vi "BMP180 Init.vi"(7 "I2C Channel":u8=1, 8 "error in (no error)":errorcluster, 9 "BMP180 Config Options":T1={"Mode"=enum."Ultra Low Power", "Cal Coefs"={"AC1"={"Addr:"=170, "Val:"=0}, "AC2"={"Addr:"=172, "Val:"=0}, "AC3"={"Addr:"=174, "Val:"=0}, "AC4"={"Addr:"=176, "Val:"=0}, "AC5"={"Addr:"=178, "Val:"=0}, "AC6"={"Addr:"=180, "Val:"=0}, "B1"={"Addr:"=182, "Val:"=0}, "B2"={"Addr:"=184, "Val:"=0}, "MB"={"Addr:"=186, "Val:"=0}, "MC"={"Addr:"=188, "Val:"=0}, "MD"={"Addr:"=190, "Val:"=0}}} {"Cal Coefs"."MD"."Val:" format="%04x"; "Cal Coefs"."MD"."Addr:" format="%02x"; "Cal Coefs"."MC"."Val:" format="%04x"; "Cal Coefs"."MC"."Addr:" format="%02x"; "Cal Coefs"."MB"."Val:" format="%04x"; "Cal Coefs"."MB"."Addr:" format="%02x"; "Cal Coefs"."B2"."Val:" format="%04x"; "Cal Coefs"."B2"."Addr:" format="%02x"; "Cal Coefs"."B1"."Val:" format="%04x"; "Cal Coefs"."B1"."Addr:" format="%02x"; "Cal Coefs"."AC6"."Val:" format="%04x"; "Cal Coefs"."AC6"."Addr:" format="%02x"; "Cal Coefs"."AC5"."Val:" format="%04x"; "Cal Coefs"."AC5"."Addr:" format="%02x"; "Cal Coefs"."AC4"."Val:" format="%04x"; "Cal Coefs"."AC4"."Addr:" format="%02x"; "Cal Coefs"."AC3"."Val:" format="%04x"; "Cal Coefs"."AC3"."Addr:" format="%02x"; "Cal Coefs"."AC2"."Val:" format="%04x"; "Cal Coefs"."AC2"."Addr:" format="%02x"; "Cal Coefs"."AC1"."Val:" format="%04x"; "Cal Coefs"."AC1"."Addr:" format="%02x"}, 10 "I2C Slave Address":u8=119 format="%.0x", 11 "LINX Resource in":T2) -> (0 "error out":errorcluster, 1 "BMP180 Config Options":T1 {"Cal Coefs"."MD"."Val:" format="%04x"; "Cal Coefs"."MD"."Addr:" format="%02x"; "Cal Coefs"."MC"."Val:" format="%04x"; "Cal Coefs"."MC"."Addr:" format="%02x"; "Cal Coefs"."MB"."Val:" format="%04x"; "Cal Coefs"."MB"."Addr:" format="%02x"; "Cal Coefs"."B2"."Val:" format="%04x"; "Cal Coefs"."B2"."Addr:" format="%02x"; "Cal Coefs"."B1"."Val:" format="%04x"; "Cal Coefs"."B1"."Addr:" format="%02x"; "Cal Coefs"."AC6"."Val:" format="%04x"; "Cal Coefs"."AC6"."Addr:" format="%02x"; "Cal Coefs"."AC5"."Val:" format="%04x"; "Cal Coefs"."AC5"."Addr:" format="%02x"; "Cal Coefs"."AC4"."Val:" format="%04x"; "Cal Coefs"."AC4"."Addr:" format="%02x"; "Cal Coefs"."AC3"."Val:" format="%04x"; "Cal Coefs"."AC3"."Addr:" format="%02x"; "Cal Coefs"."AC2"."Val:" format="%04x"; "Cal Coefs"."AC2"."Addr:" format="%02x"; "Cal Coefs"."AC1"."Val:" format="%04x"; "Cal Coefs"."AC1"."Addr:" format="%02x"}, 3 "LINX Resource out":T2)   [LabVIEW 2014]
uses:
  <vilib>/MakerHub/LINX/Private/Type Defs/LINX Ref.ctl
  <vilib>/MakerHub/LINX/Private/Type Defs/Platform.ctl
  <vilib>/MakerHub/LINX/Private/Type Defs/Interface.ctl
  <vilib>/MakerHub/LINX/Private/Device/Type Defs/LINX Device Config.ctl
  <vilib>/MakerHub/LINX/Private/Device/Type Defs/TCP Config.ctl
  <vilib>/MakerHub/LINX/Private/Device/Type Defs/Channels.ctl
  BMP180 Config Options.ctl
  <vilib>/MakerHub/LINX/Private/Local IO/LinxI2cWrite.vi
  <vilib>/MakerHub/LINX/Public/Utilities/Check Channel.vi
  <vilib>/myRIO/Instrument Drivers/Onboard IO/I2C/vis/Write.vi
  <vilib>/MakerHub/LINX/Private/Utilties/Generate Error.vi
  <vilib>/MakerHub/LINX/Private/Utilties/Channel FGVs/I2C Channels.vi
  <vilib>/Utility/error.llb/Error Cluster From Error Code.vi
  <vilib>/myRIO/Common/Instrument Driver Framework/myRIO v1.0/I2C/vis/myRIO v1.0 Write I2C.vi
  <vilib>/MakerHub/LINX/LMH-LINX.lvlib
  <vilib>/MakerHub/LINX/Private/Device/Device.lvlib
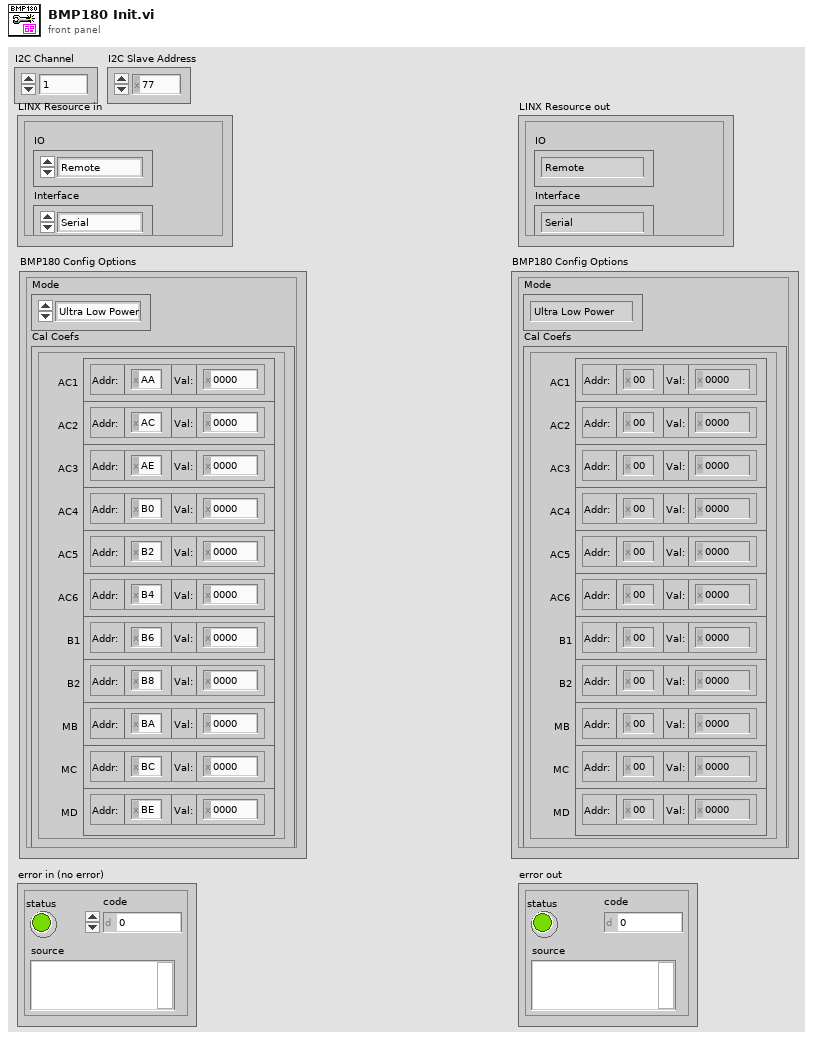
[diagram p1: front panel]
types:
  T1 = typedef "BMP180 Config Options.ctl" = cluster{"Mode":enum8{"Ultra Low Power", "Standard", "High Resolution", "Ultra High Resolution"}, "Cal Coefs":cluster{"AC1":cluster{"Addr:":u8, "Val:":u16}, "AC2":cluster{"Addr:":u8, "Val:":u16}, "AC3":cluster{"Addr:":u8, "Val:":u16}, "AC4":cluster{"Addr:":u8, "Val:":u16}, "AC5":cluster{"Addr:":u8, "Val:":u16}, "AC6":cluster{"Addr:":u8, "Val:":u16}, "B1":cluster{"Addr:":u8, "Val:":u16}, "B2":cluster{"Addr:":u8, "Val:":u16}, "MB":cluster{"Addr:":u8, "Val:":u16}, "MC":cluster{"Addr:":u8, "Val:":u16}, "MD":cluster{"Addr:":u8, "Val:":u16}}}
  T2 = typedef "LMH-LINX.lvlib/LINX Ref.ctl" = cluster{"IO":T3, "Interface":T4, "LINX Device Config":T5}
  T3 = typedef "LMH-LINX.lvlib/Platform.ctl" = enum16{"Remote", "Local"}
  T4 = typedef "LMH-LINX.lvlib/Interface.ctl" = enum16{"Serial", "TCP"}
  T5 = typedef "LMH-LINX.lvlib/Device.lvlib/LINX Device Config.ctl" = cluster{"Interface":T4, "COM Port":refnum<visa-resource-name>, "TCP Configuration":T6, "Device Family":u8, "Device ID":u8, "Device Name":string, "TCP Ref":refnum<k5>, "Channels":T7}
  T6 = typedef "LMH-LINX.lvlib/Device.lvlib/TCP Config.ctl" = cluster{"IP Address":string, "Port":u16}
  T7 = typedef "LMH-LINX.lvlib/Channels.ctl" = cluster{"DI":u8[], "DO":u8[], "AI":u8[], "AO":u8[], "PWM":u8[], "QE":u8[], "UART":u8[], "I2C 2":u8[], "SPI":u8[], "CAN":u8[], "Servo":u8[], "AI Ref (V)":dbl, "AI Resolution (Bits)":u8, "AO Ref (V)":dbl, "AO Resolution (Bits)":u8}
  T8 = cluster{"AC1":cluster{"Addr:":u8, "Val:":u16}, "AC2":cluster{"Addr:":u8, "Val:":u16}, "AC3":cluster{"Addr:":u8, "Val:":u16}, "AC4":cluster{"Addr:":u8, "Val:":u16}, "AC5":cluster{"Addr:":u8, "Val:":u16}, "AC6":cluster{"Addr:":u8, "Val:":u16}, "B1":cluster{"Addr:":u8, "Val:":u16}, "B2":cluster{"Addr:":u8, "Val:":u16}, "MB":cluster{"Addr:":u8, "Val:":u16}, "MC":cluster{"Addr:":u8, "Val:":u16}, "MD":cluster{"Addr:":u8, "Val:":u16}}
  T9 = cluster{"[0]":cluster{"Addr:":u8, "Val:":u16}, "[1]":cluster{"Addr:":u8, "Val:":u16}, "[2]":cluster{"Addr:":u8, "Val:":u16}, "[3]":cluster{"Addr:":u8, "Val:":u16}, "[4]":cluster{"Addr:":u8, "Val:":u16}, "[5]":cluster{"Addr:":u8, "Val:":u16}, "[6]":cluster{"Addr:":u8, "Val:":u16}, "[7]":cluster{"Addr:":u8, "Val:":u16}, "[8]":cluster{"Addr:":u8, "Val:":u16}, "[9]":cluster{"Addr:":u8, "Val:":u16}, "[10]":cluster{"Addr:":u8, "Val:":u16}}
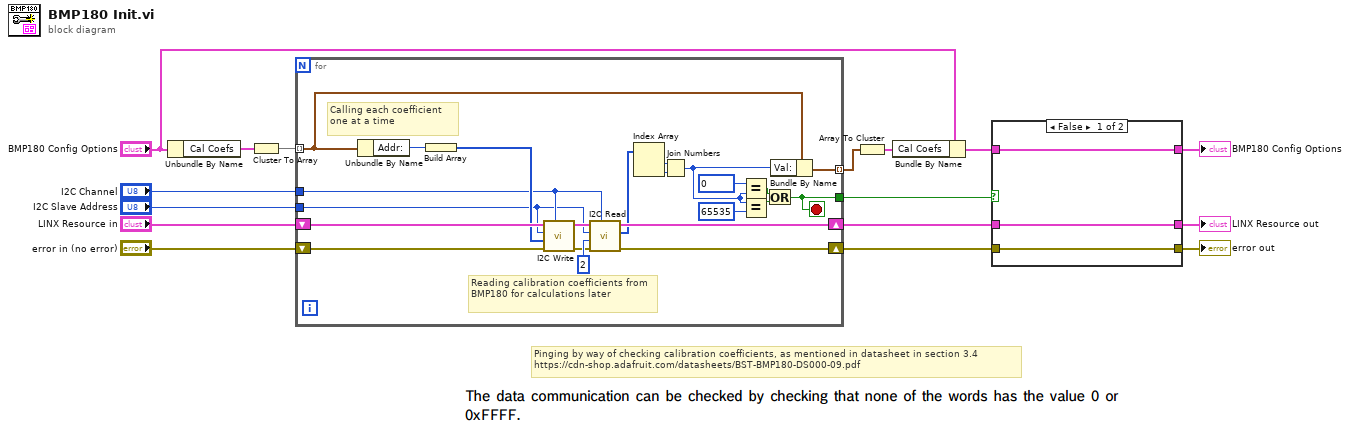
[diagram p0: block diagram]
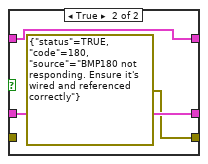
[diagram p2: hidden frame]
diagram:
  # "Pinging by way of checking calibration coefficients, as mentioned in datasheet in section 3.4\nhttps://cdn-shop.adafruit.com/datasheets/BST-BMP180-DS000-09.pdf"
  n1 = Unbundle By Name("BMP180 Config Options") -> ("Cal Coefs"=w6:T8)
  n2 = Cluster To Array(cluster=w6) -> (array=w5:cluster{"Addr:":u8, "Val:":u16}[])
  n3 = for {
    tunnel: "I2C Slave Address" -> [w17]
    tunnel: "I2C Channel" -> [w18]
    shift-right: [w37] -> w11
    shift-left: "LINX Resource in" -> [w32]
    shift-right: [w38] -> w10
    shift-left: "error in (no error)" -> [w22]
    tunnel: [w25] -> w9
    tunnel: w5 -> [w21] mode=indexing
    tunnel: [w19] -> w4 mode=indexing
    stop <- w25 stop-if-true
    # "Calling each coefficient one at a time"
    # "Reading calibration coefficients from BMP180 for calculations later"
    n4 = Unbundle By Name(w21) -> ("Addr:"=w24:u8)
    n5 = Build Array(w24) -> (w23:u8[])
    n6 = call <vilib>:"I2C Write.vi"("I2C Channel"=w18, "Error In"=w22, "Data"=w23, "I2C Slave Address (0)"=w17, "LINX Resource"=w32) -> ("Error Out"=w31:errorcluster, "LINX Resource"=w30:T2)  [unwired: 5 in]
    n7 = call <vilib>:"I2C Read.vi"("I2C Channel"=w18, "Error In"=w31, "Bytes To Read"=u8 2, "I2C Slave Address (0)"=w17, "LINX Resource"=w30) -> ("Error Out"=w38:errorcluster, "Data"=w33:u8[], "LINX Resource"=w37:T2)  [unwired: 4 in]
    n8 = Index Array(array=w33) -> (element #1=w35:u8, element #2=w34:u8)  [unwired: 2 in]
    n9 = Join Numbers(hi=w35, lo=w34) -> ((hi.lo)=w20:u16)
    n10 = Equal?(x=u16 0 ("(hi.lo)"), y=w20) -> (x = y?=w26:bool)
    n11 = Equal?(x=w20, y=u16 65535 ("(hi.lo)")) -> (x = y?=w27:bool)
    n12 = Or(x=w26, y=w27) -> (x .or. y?=w25:bool)
    n13 = Bundle By Name(cluster=w21, "Val:"=w20) -> (w19:cluster{"Addr:":u8, "Val:":u16})
  }
  n14 = Array To Cluster(array=w4) -> (cluster=w3:T9)
  n15 = Bundle By Name(cluster="BMP180 Config Options", "Cal Coefs"=w3) -> (w1:T1)
  n16 = case shown="False" w9 {
    tunnel: w11 -> [w40 w44]
    tunnel: [w40 w44] -> w13
    tunnel: w10 -> [w41 _]
    tunnel: [w41 errorcluster {"status"=TRUE, "code"=180, "source"="BMP180 not responding. Ensure it's wired and referenced correctly"} ("error constant")] -> w12
    tunnel: [w39 w42] -> w8
    tunnel: w1 -> [w39 w42]
    frame False {
    }
    frame True {
    }
  }
  "error out" <- w12
  "LINX Resource out" <- w13
  "BMP180 Config Options" <- w8
